vi "AVI Video-Write path to FG.vi"(8 "error in (no error)":errorcluster, 9 "Channel":T1, 11 "AVI2 path":path) -> (0 "error out":errorcluster)   [LabVIEW 2017]
uses:
  Typedefs/Channel Selector.ctl
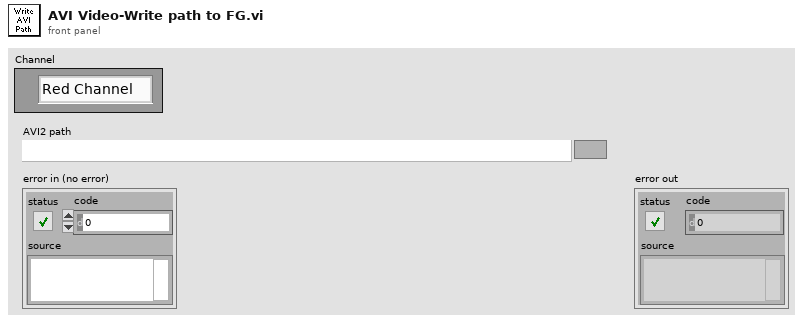
[diagram p1: front panel]
types:
  T1 = typedef "Channel Selector.ctl" = enum16{"Red Channel", "Green Channel", "Blended"}
  T2 = enum16{"Write Red AVI", "Write Green AVI", "Write AVI mode"}
  T3 = typedef "AVI Refs cluster.ctl" = cluster{"AVI2 path":path, "AVI 2 Refnum":T4, "New Image":T5, "error out":errorcluster, "Avi 1 Refnum":T6}
  T4 = typedef "IMAQ AVI2 Refnum.ctl" = refnum<k20>
  T5 = typedef "IMAQ Image.ctl" = refnum<image>
  T6 = typedef "AviRefnum.ctl" = refnum<k1>
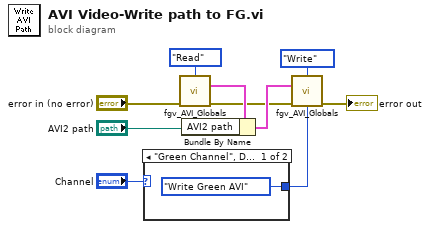
[diagram p0: block diagram]
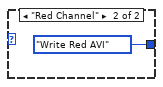
[diagram p2: hidden frame]
diagram:
  n1 = case shown="\"Green Channel\", Default" "Channel" {
    tunnel: [T2."Write Green AVI" ("Write AVI path") T2."Write Red AVI" ("Write AVI path")] -> w5
    frame "Green Channel", Default {
    }
    frame "Red Channel" {
    }
  }
  n2 = call "fgv_AVI_Globals.vi"("Function"=enum16{"Intialize", "Write", "Read", "Clear"}."Read", "error in (no error)"="error in (no error)") -> ("Red AVI"=w8:T3, "error out"=w4:errorcluster)  [unwired: 10 in, 2 out]
  n3 = Bundle By Name(cluster=w8, "AVI2 path"="AVI2 path") -> (w7:T3)
  n4 = call "fgv_AVI_Globals.vi"("Function"=enum16{"Intialize", "Write", "Read", "Clear"}."Write", "Red AVI"=w7, "error in (no error)"=w4, "\"Write\" sub function"=w5) -> ("error out"=→"error out":errorcluster)  [unwired: 8 in, 3 out]
